vi "set_query force.vi"(8 "error in (no error)":errorcluster, 9 "Query?":bool, 10 "Force Level (100 %)":u32=30 min=1 max=100 step=1, 11 "VISA resource name":refnum<visa-resource-name>) -> (0 "error out":errorcluster, 1 "Output force":string, 3 "VISA resource name out":refnum<visa-resource-name>)   [LabVIEW 2016]
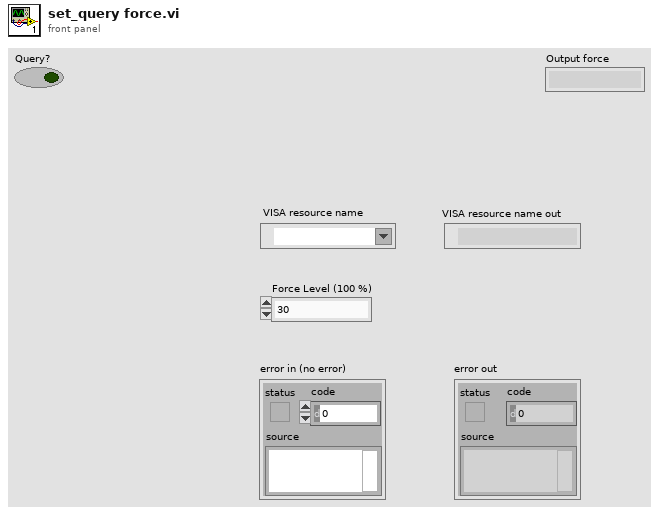
[diagram p1: front panel]
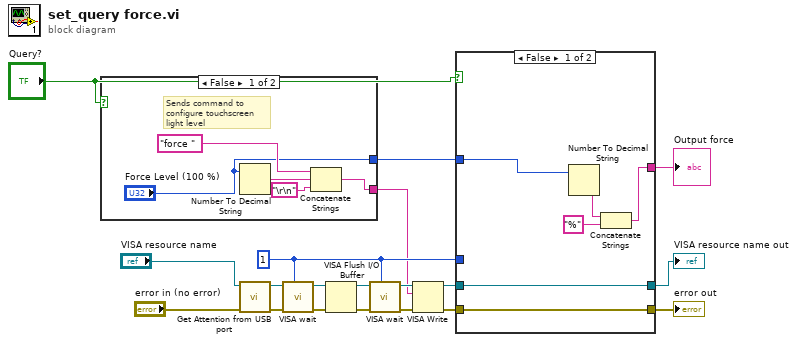
[diagram p0: block diagram]
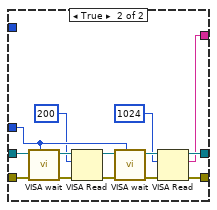
[diagram p2: hidden frame]
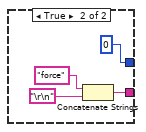
[diagram p3: hidden frame]
diagram:
  w5 = u32 1 ("milliseconds to wait")
  n1 = case shown="False" "Query?" {
    tunnel: [w21 w26] -> w4
    tunnel: ["Force Level (100 %)" u32 0 ("Force Level (100 %)")] -> w1
    frame False {
      # "Sends command to configure touchscreen light level"
      n2 = Number To Decimal String(number="Force Level (100 %)") -> (decimal integer string=w23:string)  [unwired: 1 in]
      n3 = Concatenate Strings("force " ("command"), w23, "\r\n") -> (w21:string)
    }
    frame True {
      n4 = Concatenate Strings("force" ("command"), "\r\n") -> (w26:string)
    }
  }
  n5 = call "Get Attention from USB port.vi"("error in (no error)"="error in (no error)", "VISA resource name"="VISA resource name") -> ("error out"=w16:errorcluster, "VISA resource name out"=w17:refnum<visa-resource-name>)  [unwired: 8 in]
  n6 = call <userlib>:"VISA wait.vi"("VISA resource name"=w17, "error in (no error)"=w16, "milliseconds to wait"=w5) -> ("VISA resource name out"=w14:refnum<visa-resource-name>, "error out"=w15:errorcluster)  [unwired: 6 in]
  n7 = VISA Flush I/O Buffer(VISA resource name=w14, error in (no error)=w15) -> (VISA resource name out=w9:refnum<visa-resource-name>, error out=w8:errorcluster)  [unwired: 1 in]
  n8 = call <userlib>:"VISA wait.vi"("VISA resource name"=w9, "error in (no error)"=w8, "milliseconds to wait"=w5) -> ("VISA resource name out"=w7:refnum<visa-resource-name>, "error out"=w6:errorcluster)  [unwired: 6 in]
  n9 = VISA Write(VISA resource name=w7, write buffer=w4, error in (no error)=w6) -> (VISA resource name out=w13:refnum<visa-resource-name>, error out=w12:errorcluster)  [unwired: 1 out]
  n10 = case shown="False" "Query?" {
    tunnel: w13 -> [w34 w48]
    tunnel: w12 -> [w33 w47]
    tunnel: [w34 w40] -> w11
    tunnel: [w33 w39] -> w10
    tunnel: w5 -> [_ w38]
    tunnel: [w30 w35] -> w2
    tunnel: w1 -> [w32 _]
    frame False {
      n11 = Number To Decimal String(number=w32) -> (decimal integer string=w31:string)  [unwired: 1 in]
      n12 = Concatenate Strings(w31, "%" ("string")) -> (w30:string)
    }
    frame True {
      n13 = call <userlib>:"VISA wait.vi"("VISA resource name"=w48, "error in (no error)"=w47, "milliseconds to wait"=w38) -> ("VISA resource name out"=w45:refnum<visa-resource-name>, "error out"=w46:errorcluster)  [unwired: 6 in]
      n14 = VISA Read(VISA resource name=w45, byte count=u32 200, error in (no error)=w46) -> (VISA resource name out=w44:refnum<visa-resource-name>, error out=w43:errorcluster)  [unwired: 2 out]
      n15 = call <userlib>:"VISA wait.vi"("VISA resource name"=w44, "error in (no error)"=w43, "milliseconds to wait"=w38) -> ("VISA resource name out"=w41:refnum<visa-resource-name>, "error out"=w42:errorcluster)  [unwired: 6 in]
      n16 = VISA Read(VISA resource name=w41, byte count=u32 1024, error in (no error)=w42) -> (VISA resource name out=w40:refnum<visa-resource-name>, read buffer=w35:string, error out=w39:errorcluster)  [unwired: 1 out]
    }
  }
  "VISA resource name out" <- w11
  "error out" <- w10
  "Output force" <- w2
